vi "StepperControlWavelength.vi"() -> ()   [LabVIEW 2014, in "Stepper3D.lvlib"]
uses:
  stepper3D.lvlib
  <vilib>/Utility/error.llb/DialogType.ctl
  Enums/BoundaryStatus.ctl
  <vilib>/Utility/config.llb/Read Key (Double).vi
  <vilib>/Utility/config.llb/Write Key (Double).vi
  <vilib>/Utility/config.llb/NI_LVConfig.lvlib
  array.lib/Array.lvlib
panel:
  out "St3:Right":bool
  out "St3:Left":bool
  out "St2:Right":bool
  out "St2:Left":bool
  out "St1:Right":bool
  out "St1:Left":bool
  in  "Speed":string="300"
  in  "UI:LoadConversionTables":bool
  in  "Conversion 3":path=path "C:/Users/219-PC/Dropbox/МФД/Alexandr Bogomolov/Кумарин 47/Эталон.txt"
  in  "Conversion 2":path=path "C:/Users/219-PC/Dropbox/МФД/Alexandr Bogomolov/Кумарин 47/Эталон.txt"
  in  "Conversion 1":path=path "C:/Users/219-PC/Dropbox/МФД/Alexandr Bogomolov/Кумарин 47/Решетка 3D.txt"
  out "WL:WLToStepper3":dbl[][](array[numeric])
  out "WL:WLToStepper2":dbl[][](array[numeric])=[[115.0, 0.0], [135.0, 0.0]]
  out "WL:WLToStepper1":dbl[][](array[numeric])
  in  "WL:NewValue":dbl=450.0
  in  "WL:Stop":bool
  in  "WL:SetValue":bool
  out "App:RefreshLED":bool
  in  "App:RefreshRate":u32=500 caption="Refresh every"
  in  "App:Refresh":bool
  in  "App:Disconnect":bool
  in  "App:Connect":bool
  in  "St3:SetPos":bool
  in  "St2:SetPos":bool
  in  "St1:SetPos":bool
  in  "St:Stop":bool
  in  "St3:Steps":dbl
  in  "St3:NewPosition":dbl=2605.0
  out "St3:Position":dbl=2903.0
  in  "St2:Steps":dbl
  in  "St2:NewPosition":dbl=-2500.0
  out "St2:Position":dbl=-2500.0
  in  "St:DoSteps":bool
  in  "St1:Steps":dbl
  in  "St1:NewPosition":dbl=-57680.0
  out "St1:Position":dbl=-57680.0
  in  "App:ResourceName":refnum<visa-resource-name>="COM8"
  # "ms."
  # "BOUNDARY"
  # "FUNCTIONS"
  # "POSITION"
  # "NEW POSITION"
  # "STEPS"
  # "Решетка"
  # "Фабри-Перо"
  # "Кристалл"
  # "Длина волны"
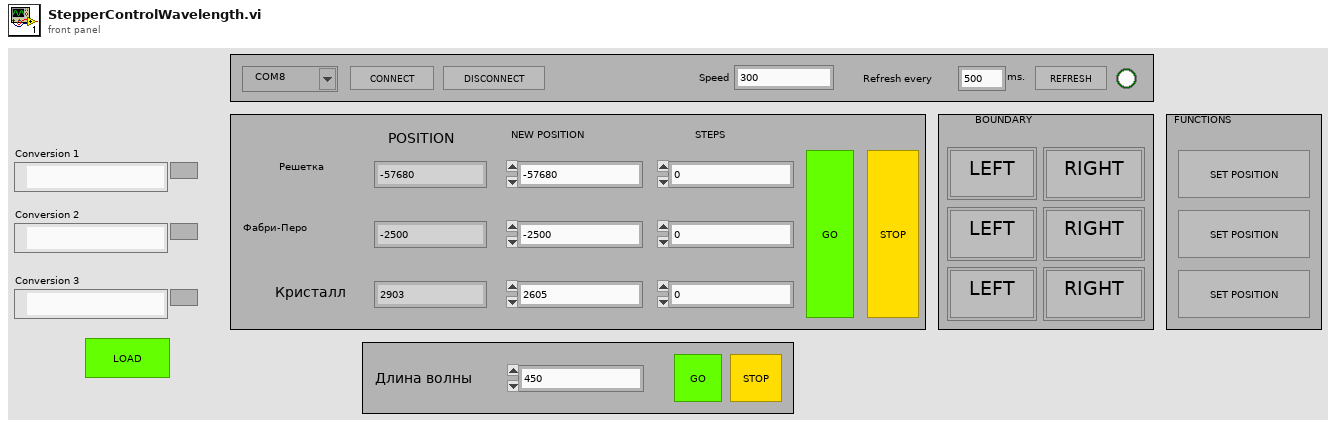
[diagram p1: front panel]
types:
  T1 = enum32{"invalid app kind", "Development System", "Run Time System", "Student Edition", "Embedded LabVIEW", "Evaluation", "Custom"}
  T2 = enum32{"Invalid", "Standard", "Closed", "Hidden", "Minimized", "Maximized"}
  T3 = typedef "stepper3D.lvlib/BoundaryStatus.ctl" = enum16{"NO BOUNDARY", "OUT OF LEFT", "OUT OF RIGHT"}
  T4 = cluster{"Core":cluster{"Current VI Reference":refnum<vi>, "Close Panel on Exit?":bool}, "VISA resource":refnum<visa-resource-name>, "App:RefreshRate":u32, "isConnected":bool, "appended path":path}
  T5 = typedef "DialogType.ctl" = u16
  T6 = cluster{"Current VI Reference":refnum<vi>, "Close Panel on Exit?":bool}
  T7 = typedef "NI_LVConfig.lvlib/Config Data RefNum.ctl" = refnum<k1>
  T8 = enum8{"Enabled", "Disabled", "Disabled and Grayed Out"}
  T9 = typedef "stepper3D.lvlib/CurrentStatus.ctl" = cluster{"desired":dbl[], "current":dbl[], "boundaries":T3[], "is running":bool}
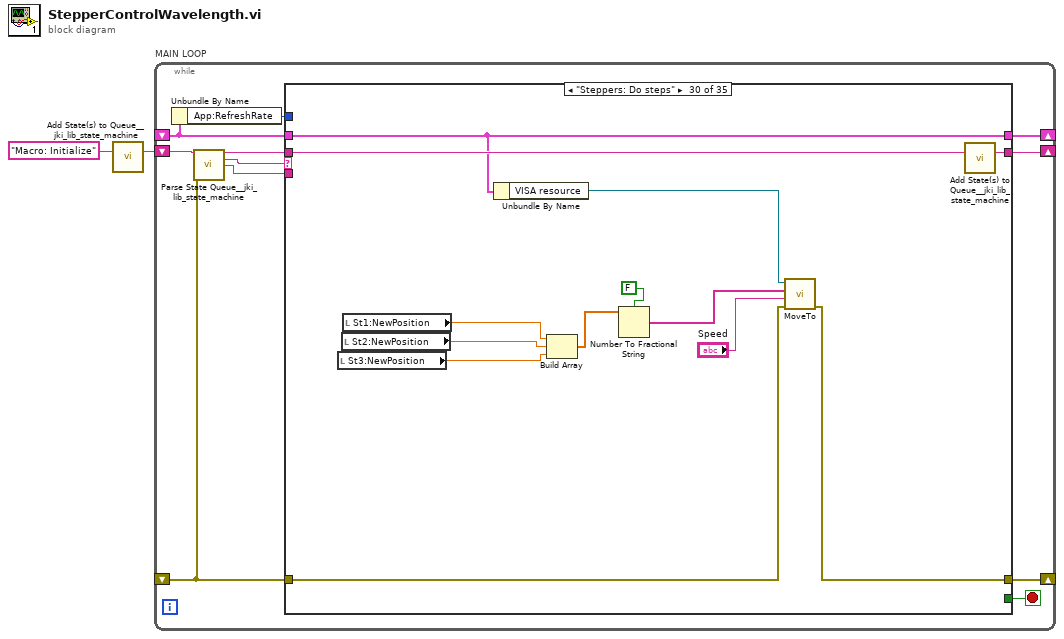
[diagram p0: block diagram]
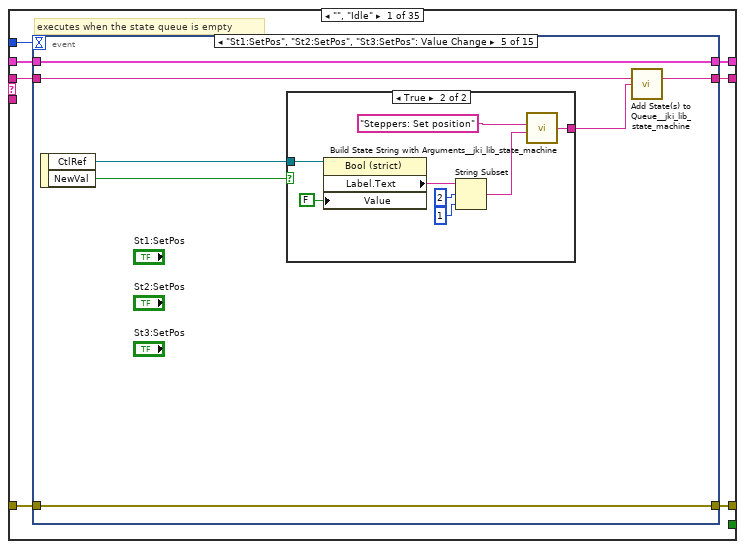
[diagram p2: hidden frame]
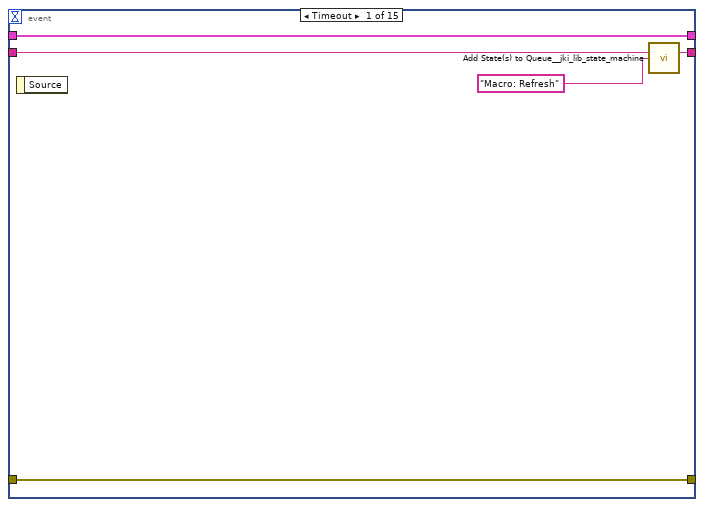
[diagram p3: hidden frame]
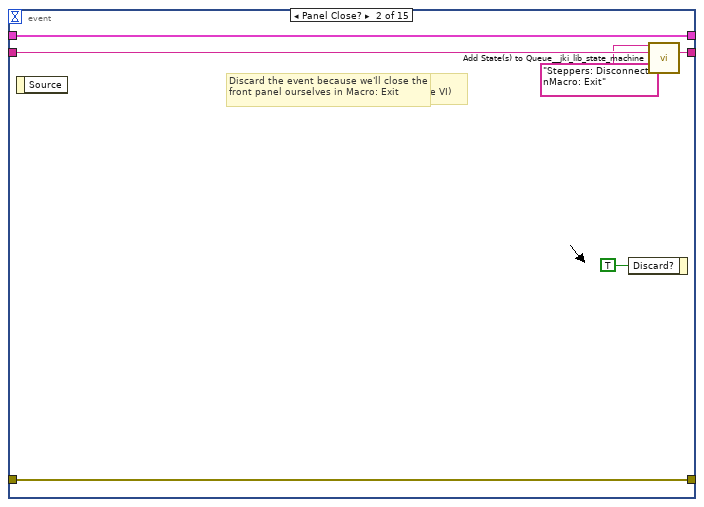
[diagram p4: hidden frame]
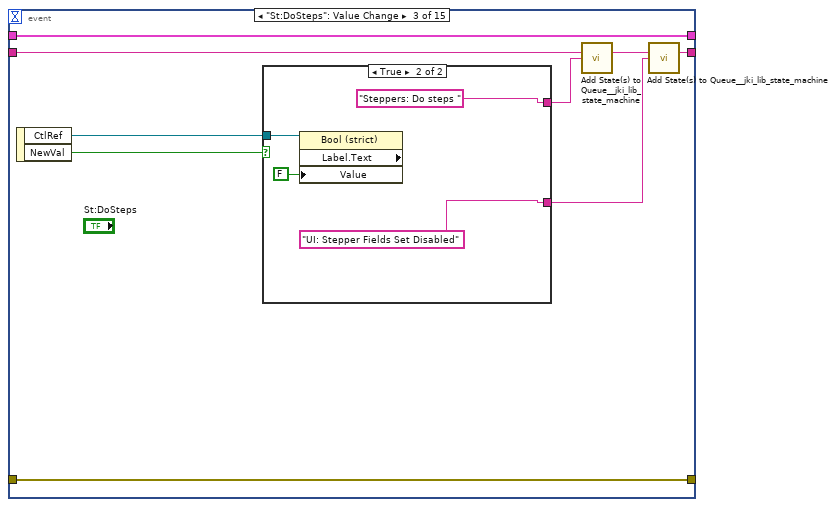
[diagram p5: hidden frame]
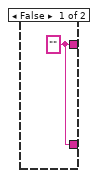
[diagram p6: hidden frame]
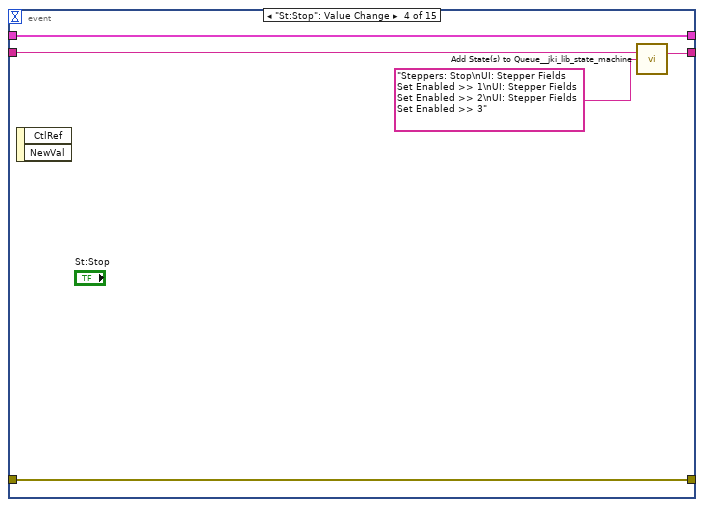
[diagram p7: hidden frame]
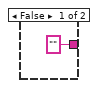
[diagram p8: hidden frame]
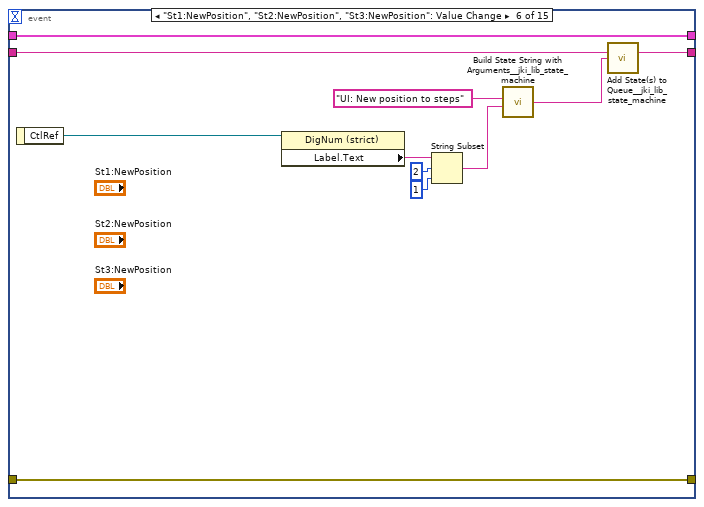
[diagram p9: hidden frame]
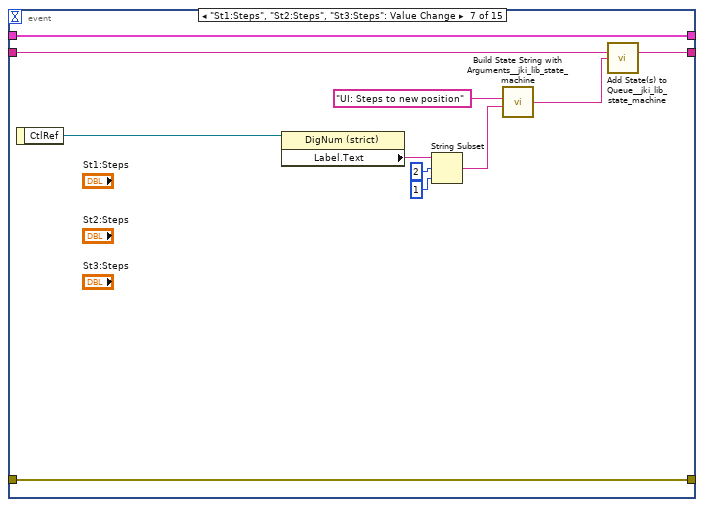
[diagram p10: hidden frame]
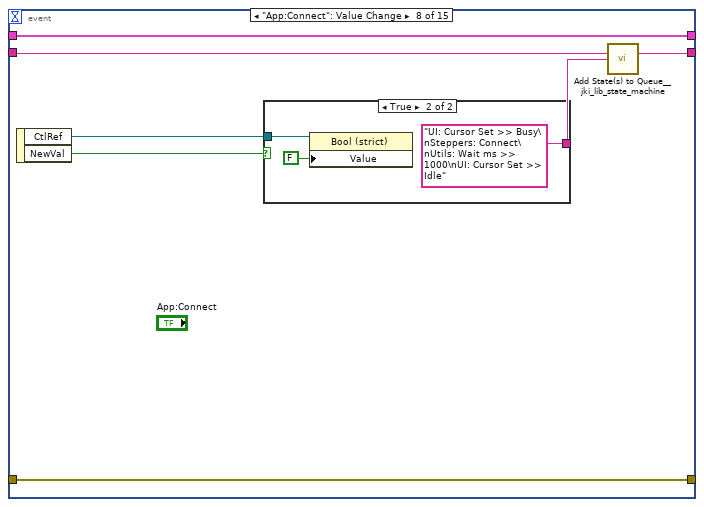
[diagram p11: hidden frame]
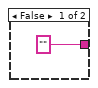
[diagram p12: hidden frame]
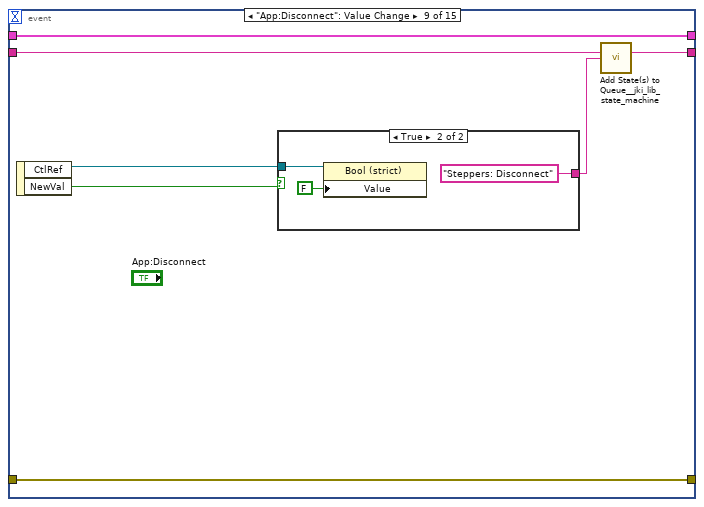
[diagram p13: hidden frame]
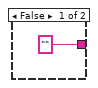
[diagram p14: hidden frame]
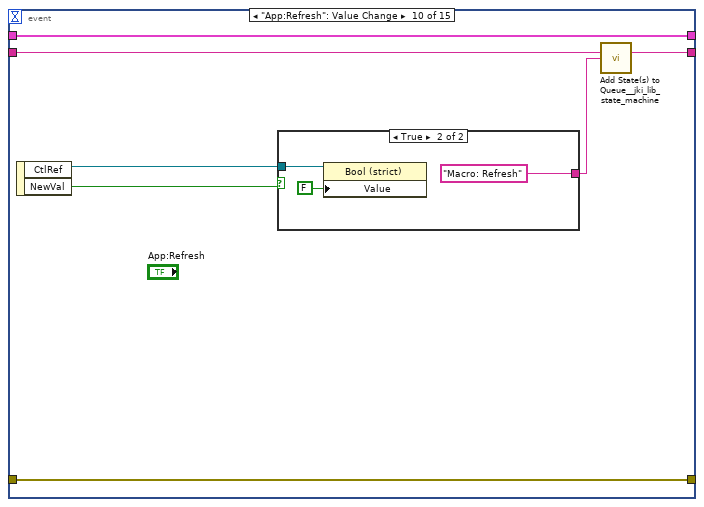
[diagram p15: hidden frame]
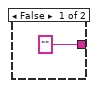
[diagram p16: hidden frame]
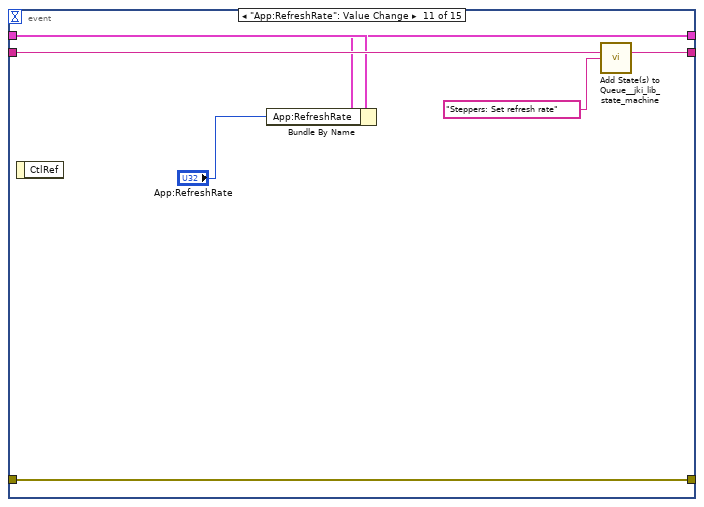
[diagram p17: hidden frame]
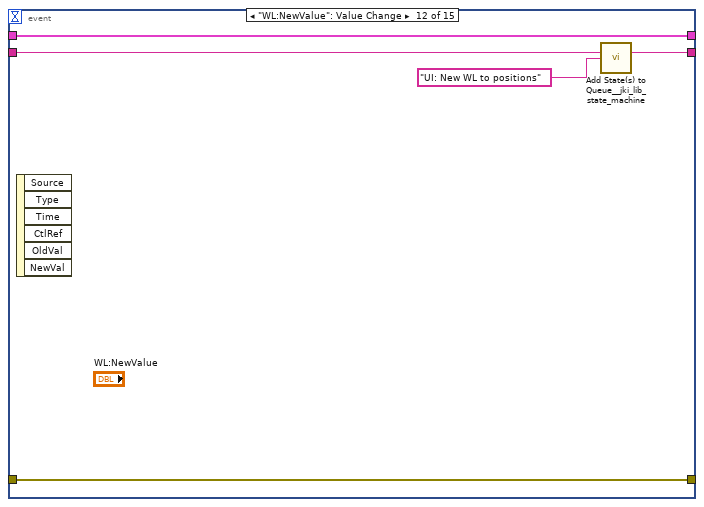
[diagram p18: hidden frame]
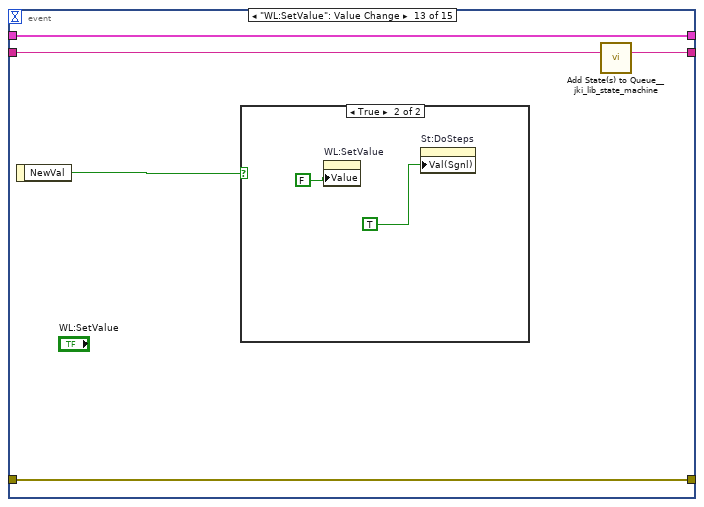
[diagram p19: hidden frame]
diagram:
  n1 = call <vilib>:"Add State(s) to Queue__jki_lib_state_machine.vi"("State(s) in (\"\")"="Macro: Initialize") -> ("States Out"=w2:string)  [unwired: 14 in]
  n2 = while "MAIN LOOP" {
    shift-right: [w7] -> _
    shift-left: _ -> [w3]
    shift-right: [w10] -> _
    shift-left: _ -> [w6]
    shift-right: [w9] -> _
    shift-left: w2 -> [w11]
    stop <- w8 stop-if-true
    n3 = Unbundle By Name(w3) -> ("App:RefreshRate"=w4:u32)
    n4 = call <vilib>:"Parse State Queue__jki_lib_state_machine.vi"("State Queue"=w11, "Error In (no error)"=w6) -> ("Remaining States"=w13:string, "Current State"=w5:string, "Arguments"=w12:string)  [unwired: 11 in]
    n5 = case shown="\"Steppers: Do steps\"" w5 {
      selector: w5 -> [_ _ w160 _ _ _ _ _ _ _ _ _ _ _ _ _ _ _ _ _ _ _ _ _ _ _ _ _ _ _ _ _ _ _ _]
      tunnel: w13 -> [w20 w159 w164 w182 w189 w194 w198 w209 w220 w239 w261 w267 w271 w276 w281 w286 w288 w307 w310 w328 w333 w340 w371 w376 w382 w394 w398 w404 w413 w429 w446 w457 w460 w527 w534]
      tunnel: w12 -> [_ _ _ _ _ _ _ _ _ _ _ _ _ _ _ _ w287 _ w311 w323 w336 w341 _ _ _ _ _ _ _ _ w442 _ _ _ w530]
      tunnel: w3 -> [w18 w156 w162 w173 w186 w192 w195 w206 _ w237 w258 w263 w268 w273 w278 w284 w290 w309 w313 w326 w337 w343 w368 w373 w379 w391 w395 w409 w412 w427 w443 w455 w465 w524 w531]
      tunnel: [w17 w157 w166 w179 errorcluster {"status"=FALSE, "code"=0, "source"=""} ("error out") w191 w196 w207 w217 w221 w259 w264 w269 w274 w279 w283 w289 w308 w312 w324 w335 w344 w369 w374 w380 w392 w396 w401 w414 w424 w441 w452 w462 w525 w532] -> w10
      tunnel: w6 -> [w16 w157 w165 w179 w185 w191 w196 w207 w217 w222 w259 w262 w269 w274 w279 w283 w289 w308 w312 w325 w335 w345 w369 w374 w380 w392 w396 w399 w415 w425 w440 w453 w463 w525 w532]
      tunnel: [w19 w158 w163 w181 w188 w193 w197 w208 w219 w238 w260 w266 w270 w275 w280 w285 w288 w307 w310 w327 w333 w340 w370 w375 w381 w393 w397 w405 w413 w428 w445 w456 w459 w526 w533] -> w9
      tunnel: [_ _ _ _ _ TRUE _ _ _ _ _ _ _ _ _ _ _ _ _ _ _ _ _ _ _ _ _ _ _ _ _ _ _ _ _] -> w8
      tunnel: [w15 w156 w162 w180 w186 w192 w195 w206 w218 w237 w258 w263 w268 w273 w278 w284 w290 w309 w313 w326 w337 w343 w368 w373 w379 w391 w395 w408 w411 w427 w443 w455 w465 w524 w531] -> w7
      tunnel: w4 -> [w14 _ _ _ _ _ _ _ _ _ _ _ _ _ _ _ _ _ _ _ _ _ _ _ _ _ _ _ _ _ _ _ _ _ _]
      frame "", "Idle" {
        # "executes when the state queue is empty"
        n6 = event shown="[4] \"St1:SetPos\", \"St2:SetPos\", \"St3:SetPos\": Value Change" {
          selector: _ -> [_ _ _ _ _ _ _ _ _ _ _ _ _ _ _]
          dyn-events: _ -> [_ _ _ _ _ _ _ _ _ _ _ _ _ _ _]
          timeout: w14 -> [_ _ _ _ _ _ _ _ _ _ _ _ _ _ _]
          tunnel: w20 -> [w25 w31 w36 w47 w53 w74 w85 w92 w102 w113 w127 w132 w137 w144 w152]
          tunnel: [w24 w30 w34 w48 w52 w73 w84 w93 w103 w114 w128 w133 w138 w145 w153] -> w19
          tunnel: w18 -> [w22 w28 w39 w50 w56 w76 w87 w94 w106 w117 w124 w130 w135 w142 w150]
          tunnel: [w23 w29 w38 w49 w55 w75 w86 w95 w100 w111 w125 w131 w136 w143 w151] -> w17
          tunnel: w16 -> [w23 w29 w38 w49 w55 w75 w86 w95 w100 w111 w125 w131 w136 w143 w151]
          tunnel: [w22 w28 w39 w50 w56 w76 w87 w94 w106 w117 w123 w130 w135 w142 w150] -> w15
          event Timeout {
            n7 = event-data() -> ()  [unwired: 1 in, 1 out]
            n8 = call <vilib>:"Add State(s) to Queue__jki_lib_state_machine.vi"("State(s) in (\"\")"=w25, "State(s) at Back (\"\")"="Macro: Refresh") -> ("States Out"=w24:string)  [unwired: 13 in]
          }
          event Panel Close? {
            # "Discard the event because we'll close the front panel ourselves in Macro: Exit"
            # "Close Panel button (pressed) Event\n(this executes Macro: Exit to terminate the VI)"
            n9 = event-data() -> ()  [unwired: 1 in, 1 out]
            n10 = event-data("Discard?"=TRUE) -> ()  [unwired: 1 in, 1 out]
            n11 = call <vilib>:"Add State(s) to Queue__jki_lib_state_machine.vi"("State(s) in Front (\"\")"="Steppers: Disconnect\nMacro: Exit", "State(s) in (\"\")"=w31) -> ("States Out"=w30:string)  [unwired: 13 in]
          }
          event "St:DoSteps": Value Change {
            n12 = event-data() -> ("CtlRef"=w40:refnum<vi>, "NewVal"=w37:bool)  [unwired: 1 in]
            n13 = case shown="True" w37 {
              tunnel: w40 -> [_ w45]
              tunnel: [w41 "Steppers: Do steps "] -> w35
              tunnel: [w41 "UI: Stepper Fields Set Disabled" ("State")] -> w32
              frame False {
                w41 = "" ("State with Arguments")
              }
              frame True {
                n14 = property class="Bool (strict)" props=["Label", "Text", "Value"](reference=w45, "Value"=FALSE) -> ()  [unwired: 1 in, 3 out]
              }
            }
            n15 = call <vilib>:"Add State(s) to Queue__jki_lib_state_machine.vi"("State(s) in (\"\")"=w36, "State(s) at Back (\"\")"=w35) -> ("States Out"=w33:string)  [unwired: 13 in]
            n16 = call <vilib>:"Add State(s) to Queue__jki_lib_state_machine.vi"("State(s) in (\"\")"=w33, "State(s) at Back (\"\")"=w32) -> ("States Out"=w34:string)  [unwired: 13 in]
          }
          event "St:Stop": Value Change {
            n17 = event-data() -> ()  [unwired: 1 in, 2 out]
            n18 = call <vilib>:"Add State(s) to Queue__jki_lib_state_machine.vi"("State(s) in (\"\")"=w47, "State(s) at Back (\"\")"="Steppers: Stop\nUI: Stepper Fields Set Enabled >> 1\nUI: Stepper Fields Set Enabled >> 2\nUI: Stepper Fields Set Enabled >> 3" ("State")) -> ("States Out"=w48:string)  [unwired: 13 in]
          }
          event "St1:SetPos", "St2:SetPos", "St3:SetPos": Value Change {
            n19 = event-data() -> ("CtlRef"=w57:refnum<vi>, "NewVal"=w54:bool)  [unwired: 1 in]
            n20 = case shown="True" w54 {
              tunnel: w57 -> [_ w66]
              tunnel: ["" ("State with Arguments") w60] -> w51
              frame False {
              }
              frame True {
                n21 = property class="Bool (strict)"(reference=w66, "Value"=FALSE) -> ("Label.Text"=w63:string)  [unwired: 1 in, 2 out]
                n22 = String Subset(string=w63, offset (0)=2, length (rest)=1 ("length (rest)")) -> (substring=w61:string)
                n23 = call <vilib>:"Build State String with Arguments__jki_lib_state_machine.vi"("Arguments (\"\")"=w61, "State"="Steppers: Set position") -> ("State with Arguments"=w60:string)  [unwired: 4 in]
              }
            }
            n24 = call <vilib>:"Add State(s) to Queue__jki_lib_state_machine.vi"("State(s) in (\"\")"=w53, "State(s) at Back (\"\")"=w51) -> ("States Out"=w52:string)  [unwired: 13 in]
          }
          event "St1:NewPosition", "St2:NewPosition", "St3:NewPosition": Value Change {
            n25 = event-data() -> ("CtlRef"=w77:refnum<vi>)  [unwired: 1 in]
            n26 = property class="DigNum (strict)"(reference=w77) -> ("Label.Text"=w69:string)  [unwired: 1 in, 2 out]
            n27 = String Subset(string=w69, offset (0)=2, length (rest)=1 ("length (rest)")) -> (substring=w67:string)
            n28 = call <vilib>:"Build State String with Arguments__jki_lib_state_machine.vi"("Arguments (\"\")"=w67, "State"="UI: New position to steps") -> ("State with Arguments"=w72:string)  [unwired: 4 in]
            n29 = call <vilib>:"Add State(s) to Queue__jki_lib_state_machine.vi"("State(s) in (\"\")"=w74, "State(s) at Back (\"\")"=w72) -> ("States Out"=w73:string)  [unwired: 13 in]
          }
          event "St1:Steps", "St2:Steps", "St3:Steps": Value Change {
            n30 = event-data() -> ("CtlRef"=w88:refnum<vi>)  [unwired: 1 in]
            n31 = property class="DigNum (strict)"(reference=w88) -> ("Label.Text"=w80:string)  [unwired: 1 in, 2 out]
            n32 = String Subset(string=w80, offset (0)=2, length (rest)=1 ("length (rest)")) -> (substring=w78:string)
            n33 = call <vilib>:"Build State String with Arguments__jki_lib_state_machine.vi"("Arguments (\"\")"=w78, "State"="UI: Steps to new position") -> ("State with Arguments"=w83:string)  [unwired: 4 in]
            n34 = call <vilib>:"Add State(s) to Queue__jki_lib_state_machine.vi"("State(s) in (\"\")"=w85, "State(s) at Back (\"\")"=w83) -> ("States Out"=w84:string)  [unwired: 13 in]
          }
          event "App:Connect": Value Change {
            n35 = event-data() -> ("CtlRef"=w91:refnum<vi>, "NewVal"=w90:bool)  [unwired: 1 in]
            n36 = case shown="True" w90 {
              tunnel: w91 -> [_ w99]
              tunnel: ["" "UI: Cursor Set >> Busy\nSteppers: Connect\nUtils: Wait ms >> 1000\nUI: Cursor Set >> Idle"] -> w89
              frame False {
              }
              frame True {
                n37 = property class="Bool (strict)"(reference=w99, "Value"=FALSE) -> ()  [unwired: 1 in, 2 out]
              }
            }
            n38 = call <vilib>:"Add State(s) to Queue__jki_lib_state_machine.vi"("State(s) in (\"\")"=w92, "State(s) at Back (\"\")"=w89) -> ("States Out"=w93:string)  [unwired: 13 in]
          }
          event "App:Disconnect": Value Change {
            n39 = event-data() -> ("CtlRef"=w105:refnum<vi>, "NewVal"=w104:bool)  [unwired: 1 in]
            n40 = case shown="True" w104 {
              tunnel: w105 -> [_ w110]
              tunnel: ["" "Steppers: Disconnect"] -> w101
              frame False {
              }
              frame True {
                n41 = property class="Bool (strict)"(reference=w110, "Value"=FALSE) -> ()  [unwired: 1 in, 2 out]
              }
            }
            n42 = call <vilib>:"Add State(s) to Queue__jki_lib_state_machine.vi"("State(s) in (\"\")"=w102, "State(s) at Back (\"\")"=w101) -> ("States Out"=w103:string)  [unwired: 13 in]
          }
          event "App:Refresh": Value Change {
            n43 = event-data() -> ("CtlRef"=w116:refnum<vi>, "NewVal"=w115:bool)  [unwired: 1 in]
            n44 = case shown="True" w115 {
              tunnel: w116 -> [_ w121]
              tunnel: ["" "Macro: Refresh"] -> w112
              frame False {
              }
              frame True {
                n45 = property class="Bool (strict)"(reference=w121, "Value"=FALSE) -> ()  [unwired: 1 in, 2 out]
              }
            }
            n46 = call <vilib>:"Add State(s) to Queue__jki_lib_state_machine.vi"("State(s) in (\"\")"=w113, "State(s) at Back (\"\")"=w112) -> ("States Out"=w114:string)  [unwired: 13 in]
          }
          event "App:RefreshRate": Value Change {
            n47 = event-data() -> ()  [unwired: 1 in, 1 out]
            n48 = Bundle By Name(cluster=w124, "App:RefreshRate"="App:RefreshRate") -> (w123:T4)
            n49 = call <vilib>:"Add State(s) to Queue__jki_lib_state_machine.vi"("State(s) in (\"\")"=w127, "State(s) at Back (\"\")"="Steppers: Set refresh rate") -> ("States Out"=w128:string)  [unwired: 13 in]
          }
          event "WL:NewValue": Value Change {
            n50 = event-data() -> ()  [unwired: 1 in, 6 out]
            n51 = call <vilib>:"Add State(s) to Queue__jki_lib_state_machine.vi"("State(s) in (\"\")"=w132, "State(s) at Back (\"\")"="UI: New WL to positions" ("State(s) at Back (\"\")")) -> ("States Out"=w133:string)  [unwired: 13 in]
          }
          event "WL:SetValue": Value Change {
            n52 = event-data() -> ("NewVal"=w134:bool)  [unwired: 1 in]
            n53 = case shown="True" w134 {
              frame False {
              }
              frame True {
                n54 = property on="WL:SetValue" class="Bool (strict)"("Value"=FALSE ("WL:SetValue")) -> ()  [unwired: 2 in, 2 out]
                n55 = property on="St:DoSteps" class="Bool (strict)"("Val(Sgnl)"=TRUE) -> ()  [unwired: 2 in, 2 out]
              }
            }
            n56 = call <vilib>:"Add State(s) to Queue__jki_lib_state_machine.vi"("State(s) in (\"\")"=w137) -> ("States Out"=w138:string)  [unwired: 14 in]
          }
          event "WL:Stop": Value Change {
            n57 = event-data() -> ("NewVal"=w141:bool)  [unwired: 1 in]
            n58 = case shown="True" w141 {
              frame False {
              }
              frame True {
                n59 = property on="WL:Stop" class="Bool (strict)"("Value"=FALSE ("WL:Stop")) -> ()  [unwired: 2 in, 2 out]
                n60 = property on="St:Stop" class="Bool (strict)"("Val(Sgnl)"=TRUE) -> ()  [unwired: 2 in, 2 out]
              }
            }
            n61 = call <vilib>:"Add State(s) to Queue__jki_lib_state_machine.vi"("State(s) in (\"\")"=w144) -> ("States Out"=w145:string)  [unwired: 14 in]
          }
          event "UI:LoadConversionTables": Value Change {
            n62 = event-data() -> ("NewVal"=w149:bool)  [unwired: 1 in]
            n63 = case shown="True" w149 {
              tunnel: [_ "Data: Load Conversion Files"] -> w148
              frame False {
              }
              frame True {
                n64 = property on="UI:LoadConversionTables" class="Bool (strict)"("Value"=FALSE) -> ()  [unwired: 2 in, 2 out]
              }
            }
            n65 = call <vilib>:"Add State(s) to Queue__jki_lib_state_machine.vi"("State(s) in (\"\")"=w152, "State(s) at Back (\"\")"=w148) -> ("States Out"=w153:string)  [unwired: 13 in]
          }
        }
      }
      frame "---------- Core ----------" {
        # "Do not put any code in this frame.\n(it is a separator no-op)"
        n66 = call <vilib>:"Add State(s) to Queue__jki_lib_state_machine.vi"("State(s) in (\"\")"=w159) -> ("States Out"=w158:string)  [unwired: 14 in]
      }
      frame Default {
        w169 = 42 items=["No error", "Argument error", "Memory is full", "Out of zone", "End of file", "File already open", "Generic file I/O error", "File not found", "File permission error", "Disk is full", "Duplicate path", "Too many files open", "System feature not enabled", "Resource file not found", "Cannot add resource", "Resource not found", "Image not found", "Image memory error", "Pen does not exist", "Config type invalid", "Config token not found", "Config parse error", "Config memory error", "Bad external code format", "Bad external code offset", "External code not present", "Null window", "Destroy window error", "Null menu", "Print aborted", "Bad print record", "Print driver error", "Windows error during printing", "Memory error during printing", "Print dialog error", "Generic print error", "Invalid device refnum", "Device not found", "Device parameter error", "Device unit error", "Cannot open device", "Device call aborted", "Generic error", "Cancelled by user", "Object ID too low", "Object ID too high", "Object not in heap", "Unknown heap", "Unknown object (invalid DefProc)", "Unknown object (DefProc not in table)", "Message out of range", "Invalid (null) method", "Unknown message", "Manager call not supported", "Bad address", "Network operation in progress", "Network operation timed out", "Connection is busy", "Network attribute not supported", "Network error", "Address in use", "System out of memory", "Connection aborted", "Connection refused", "Not connected", "Already connected", "Connection closed", "Initialization error (interapplication manager)", "Bad occurrence", "Wait on unbound occurrence handler", "Occurrence queue overflow", "Datalog type conflict", "Unused", "Unrecognized type (interapplication manager)", "Memory corrupt", "Failed to make temporary DLL", "Old CIN version", "Drag socket not found", "Failed to load drop-object", "Failed to register OLE object", "Failed to release OLE object", "Format specifier type mismatch", "Unknown format specifier", "Too few format specifiers", "Too many format specifiers", "Scan failed", "Newer CIN version", "Error converting to variant", "Runtime menu error", "Password tampered", "Variant attribute not found", "Incompatible variant data type", "Event data is not available", "Event Store is not present", "Occurrence is not found", "Event Queue is not created", "Event info is not available", "Refnum passed is NULL", "Error retrieving Class GUID", "Error retrieving CoClass GUID", "Error retrieving TypeLib GUID.", "Bad built application magic bytes.", "Specific driver is different from the specific driver associated with the Logical Name.", "There is no session opened to the class driver.", "Max Error", "MAX - Error with config objects", "MAX - Error loading configuration", "MAX - Group not supported"]
        # "Current State"
        # "Handle mistyped state name (developer tool)"
        n67 = Format Into String(format string="Software Exception: Unhandled State \"%s\"." ("message"), error in=w165, w160) -> (resulting string=w168:string, error out=w167:errorcluster)  [unwired: 1 in]
        n68 = call <vilib>:"Error Cluster From Error Code.vi"("show call chain? (False)"=TRUE, "error in (no error)"=w167, "error message (\"\")"=w168, "error code (0)"=w169) -> ("error out"=w166:errorcluster)  [unwired: 5 in]
        n69 = call <vilib>:"Add State(s) to Queue__jki_lib_state_machine.vi"("State(s) in (\"\")"=w164) -> ("States Out"=w163:string)  [unwired: 14 in]
      }
      frame "Initialize Core Data" {
        # "originally closed?"
        # "exe?"
        # "If panel starts closed or is an EXE, then close it when we exit"
        n70 = property class="VI"() -> ("Front Panel.Open"=w178:bool)  [unwired: 2 in, 2 out]
        n71 = property class="App"() -> ("App.Kind"=w177:T1)  [unwired: 2 in, 2 out]
        n72 = control-ref of="Current VI Reference"() -> (w171:refnum<vi>)
        n73 = Not(x=w178) -> (.not. x?=w175:bool)
        n74 = Equal?(x=w177, y=T1."Run Time System" ("Application:Kind")) -> (x = y?=w174:bool)
        n75 = Or(x=w175, y=w174) -> (x .or. y?=w172:bool)
        n76 = Bundle By Name(cluster=w173, "Core.Current VI Reference"=w171, "Core.Close Panel on Exit?"=w172) -> (w180:T4)
        n77 = call <vilib>:"Add State(s) to Queue__jki_lib_state_machine.vi"("State(s) in (\"\")"=w182) -> ("States Out"=w181:string)  [unwired: 14 in]
      }
      frame "Error Handler" {
        w183 = T5 2 items=["no dialog", "OK message", "continue or stop message", "OK message + warnings", "continue/stop + warnings"] ("type of dialog (OK msg:1)")
        # "Unhandled Error -- Display it"
        # "Handle any errors here.\nYou can also output any states to clean-up after errors occur"
        # "Clear error"
        n78 = call <vilib>:"General Error Handler.vi"("type of dialog (OK msg:1)"=w183, "error in (no error)"=w185) -> ()  [unwired: 9 in, 5 out]
        n79 = call <vilib>:"Add State(s) to Queue__jki_lib_state_machine.vi"("State(s) in Front (\"\")"="// Post Error States", "State(s) in (\"\")"=w189) -> ("States Out"=w188:string)  [unwired: 13 in]
      }
      frame "Exit" {
        n80 = call <vilib>:"Add State(s) to Queue__jki_lib_state_machine.vi"("State(s) in (\"\")"=w194) -> ("States Out"=w193:string)  [unwired: 14 in]
      }
      frame "---------- Data ----------" {
        # "Do not put any code in this frame.\n(It is a separator no-op. You can make a copy of this frame to create a new Data frame)"
        n81 = call <vilib>:"Add State(s) to Queue__jki_lib_state_machine.vi"("State(s) in (\"\")"=w198) -> ("States Out"=w197:string)  [unwired: 14 in]
      }
      frame "Data: Load Conversion Files" {
        n82 = call "readArrayFromFile.vi"("file"="Conversion 1") -> ("array"=→"WL:WLToStepper1":dbl[][])  [unwired: 1 in, 1 out]
        n83 = call "readArrayFromFile.vi"("file"="Conversion 2") -> ("array"=→"WL:WLToStepper2":dbl[][])  [unwired: 1 in, 1 out]
        n84 = call "readArrayFromFile.vi"("file"="Conversion 3") -> ("array"=→"WL:WLToStepper3":dbl[][])  [unwired: 1 in, 1 out]
        n85 = call <vilib>:"Add State(s) to Queue__jki_lib_state_machine.vi"("State(s) in (\"\")"=w209, "State(s) at Back (\"\")"="UI: New WL to positions" ("State(s) at Back (\"\")")) -> ("States Out"=w208:string)  [unwired: 13 in]
      }
      frame "Data: Initialize" {
        w214 = FALSE  # isConnected
        w215 = refnum<visa-resource-name> refnum  # VISA resource
        w216 = T6 {"Current VI Reference"=refnum, "Close Panel on Exit?"=FALSE}  # Core
        n86 = local read "App:RefreshRate"() -> (w213:u32)
        n87 = call <vilib>:"Application Directory.vi"() -> ("Application Directory"=w212:path)
        n88 = Build Path(base path=w212, name or relative path="steppers.config") -> (appended path=w210:path)
        n89 = Bundle("Core"=w216, "VISA resource"=w215, "App:RefreshRate"=w213, "isConnected"=w214, "appended path"=w210) -> (w218:T4)  [unwired: 1 in]
        n90 = call <vilib>:"Add State(s) to Queue__jki_lib_state_machine.vi"("State(s) in (\"\")"=w220) -> ("States Out"=w219:string)  [unwired: 14 in]
      }
      frame "Data: Read Config" {
        n91 = Unbundle By Name(w237) -> ("appended path"=w224:path)
        n92 = call <vilib>:"Open Config Data.vi"("error in (no error)"=w222, "configuration file path"=w224) -> ("error out"=w221:errorcluster, "refnum"=w223:T7)  [unwired: 7 in, 1 out]
        n93 = call-poly <vilib>:"Read Key.vi"("section"="current values", "key"="wavelength", "refnum"=w223) -> ("value"=w228:dbl)  [unwired: 5 in, 3 out]
        n94 = call-poly <vilib>:"Read Key.vi"("section"="current values", "key"="stepper1", "refnum"=w223) -> ("value"=w227:dbl)  [unwired: 5 in, 3 out]
        n95 = call-poly <vilib>:"Read Key.vi"("section"="current values", "key"="stepper2", "refnum"=w223) -> ("value"=w226:dbl)  [unwired: 5 in, 3 out]
        n96 = call-poly <vilib>:"Read Key.vi"("section"="current values", "key"="stepper3", "refnum"=w223) -> ("value"=w225:dbl)  [unwired: 5 in, 3 out]
        n97 = local write "WL:NewValue"(w228) -> ()
        n98 = local write "St1:NewPosition"(w227) -> ()
        n99 = local write "St2:NewPosition"(w226) -> ()
        n100 = local write "St3:NewPosition"(w225) -> ()
        n101 = call <vilib>:"Add State(s) to Queue__jki_lib_state_machine.vi"("State(s) in (\"\")"=w239) -> ("States Out"=w238:string)  [unwired: 14 in]
      }
      frame "Data: Write Config" {
        n102 = Unbundle By Name(w258) -> ("appended path"=w242:path)
        n103 = local read "St1:Position"() -> (w248:dbl)
        n104 = local read "WL:NewValue"() -> (w249:dbl)
        n105 = local read "St2:Position"() -> (w247:dbl)
        n106 = local read "St3:Position"() -> (w246:dbl)
        n107 = call <vilib>:"Open Config Data.vi"("configuration file path"=w242) -> ("refnum"=w241:T7)  [unwired: 8 in, 2 out]
        n108 = call-poly <vilib>:"Write Key.vi"("section"="current values", "value"=w249, "key"="wavelength", "refnum"=w241) -> ("refnum out"=w245:T7)  [unwired: 5 in, 2 out]
        n109 = call-poly <vilib>:"Write Key.vi"("section"="current values", "value"=w248, "key"="stepper1", "refnum"=w245) -> ("refnum out"=w244:T7)  [unwired: 5 in, 2 out]
        n110 = call-poly <vilib>:"Write Key.vi"("section"="current values", "value"=w247, "key"="stepper2", "refnum"=w244) -> ("refnum out"=w243:T7)  [unwired: 5 in, 2 out]
        n111 = call-poly <vilib>:"Write Key.vi"("section"="current values", "value"=w246, "key"="stepper3", "refnum"=w243) -> ("refnum out"=w240:T7)  [unwired: 5 in, 2 out]
        n112 = call <vilib>:"Close Config Data.vi"("refnum"=w240) -> ()  [unwired: 9 in, 2 out]
        n113 = call <vilib>:"Add State(s) to Queue__jki_lib_state_machine.vi"("State(s) in (\"\")"=w261) -> ("States Out"=w260:string)  [unwired: 14 in]
      }
      frame "Data: Cleanup" {
        n114 = Unbundle By Name(w263) -> ("Core.Current VI Reference"=w265:refnum<vi>)
        n115 = Close Reference(reference=w265, error in (no error)=w262) -> (error out=w264:errorcluster)
        n116 = call <vilib>:"Add State(s) to Queue__jki_lib_state_machine.vi"("State(s) in (\"\")"=w267) -> ("States Out"=w266:string)  [unwired: 14 in]
      }
      frame "---------- UI ----------" {
        # "Do not put any code in this frame.\n(It is a separator no-op. You can make a copy of this frame to create a new UI frame)"
        n117 = call <vilib>:"Add State(s) to Queue__jki_lib_state_machine.vi"("State(s) in (\"\")"=w271) -> ("States Out"=w270:string)  [unwired: 14 in]
      }
      frame "UI: Stepper Fields Set Enabled" {
        w272 = T8."Enabled" ("Disabled")
        # "Set Stepper Fields state .\n(Usage: \"UI: Stepper Fields Set Enabled >> 'Stepper Number'\")"
        n118 = property on="St1:NewPosition" class="DigNum (strict)"("DisabledEnum"=w272) -> ()  [unwired: 2 in, 2 out]
        n119 = property on="St2:NewPosition" class="DigNum (strict)"("DisabledEnum"=w272) -> ()  [unwired: 2 in, 2 out]
        n120 = property on="St1:Steps" class="DigNum (strict)"("DisabledEnum"=w272) -> ()  [unwired: 2 in, 2 out]
        n121 = property on="St2:Steps" class="DigNum (strict)"("DisabledEnum"=w272) -> ()  [unwired: 2 in, 2 out]
        n122 = property on="St3:NewPosition" class="DigNum (strict)"("DisabledEnum"=w272) -> ()  [unwired: 2 in, 2 out]
        n123 = property on="St3:Steps" class="DigNum (strict)"("DisabledEnum"=w272) -> ()  [unwired: 2 in, 2 out]
        n124 = property on="St:DoSteps" class="Bool (strict)"("DisabledEnum"=w272) -> ()  [unwired: 2 in, 2 out]
        n125 = call <vilib>:"Add State(s) to Queue__jki_lib_state_machine.vi"("State(s) in (\"\")"=w276) -> ("States Out"=w275:string)  [unwired: 14 in]
      }
      frame "UI: Stepper Fields Set Disabled" {
        w277 = T8."Disabled and Grayed Out" ("Disabled")
        # "Set Stepper Fields state .\n(Usage: \"UI: Stepper Fields Set Enabled >> 'Stepper Number'\")"
        n126 = property on="St1:NewPosition" class="DigNum (strict)"("DisabledEnum"=w277) -> ()  [unwired: 2 in, 2 out]
        n127 = property on="St1:Steps" class="DigNum (strict)"("DisabledEnum"=w277) -> ()  [unwired: 2 in, 2 out]
        n128 = property on="St2:NewPosition" class="DigNum (strict)"("DisabledEnum"=w277) -> ()  [unwired: 2 in, 2 out]
        n129 = property on="St2:Steps" class="DigNum (strict)"("DisabledEnum"=w277) -> ()  [unwired: 2 in, 2 out]
        n130 = property on="St3:NewPosition" class="DigNum (strict)"("DisabledEnum"=w277) -> ()  [unwired: 2 in, 2 out]
        n131 = property on="St3:Steps" class="DigNum (strict)"("DisabledEnum"=w277) -> ()  [unwired: 2 in, 2 out]
        n132 = property on="St:DoSteps" class="Bool (strict)"("DisabledEnum"=w277) -> ()  [unwired: 2 in, 2 out]
        n133 = call <vilib>:"Add State(s) to Queue__jki_lib_state_machine.vi"("State(s) in (\"\")"=w281) -> ("States Out"=w280:string)  [unwired: 14 in]
      }
      frame "UI: Initialize" {
        n134 = call <vilib>:"Add State(s) to Queue__jki_lib_state_machine.vi"("State(s) in Front (\"\")"="UI: Stepper Fields Set Enabled" ("State(s) in Front (\"\")"), "State(s) in (\"\")"=w286) -> ("States Out"=w285:string)  [unwired: 13 in]
      }
      frame "UI: Steps to new position" {
        n135 = case shown="\"3\"" w287 {
          frame "1" {
            n136 = local read "St1:Position"() -> (w293:dbl)
            n137 = local read "St1:Steps"() -> (w292:dbl)
            n138 = Add(x=w293, y=w292) -> (x+y=w291:dbl)
            n139 = local write "St1:NewPosition"(w291) -> ()
          }
          frame "2" {
            n140 = local read "St2:Position"() -> (w296:dbl)
            n141 = local read "St2:Steps"() -> (w295:dbl)
            n142 = Add(x=w296, y=w295) -> (x+y=w294:dbl)
            n143 = local write "St2:NewPosition"(w294) -> ()
          }
          frame "3" {
            n144 = local read "St3:Position"() -> (w299:dbl)
            n145 = local read "St3:Steps"() -> (w298:dbl)
            n146 = Add(x=w299, y=w298) -> (x+y=w297:dbl)
            n147 = local write "St3:NewPosition"(w297) -> ()
          }
          frame Default {
          }
        }
      }
      frame "UI: New WL to positions" {
        n148 = local read "WL:WLToStepper1"() -> (w306:dbl[][])
        n149 = local read "WL:WLToStepper2"() -> (w304:dbl[][])
        n150 = local read "WL:WLToStepper3"() -> (w305:dbl[][])
        n151 = property on="WL:NewValue" class="DigNum (strict)"() -> ("Value"=w300:dbl)  [unwired: 2 in, 2 out]
        n152 = call "GetNearestValue.vi"("Value"=w300, "Array"=w306) -> ("Nearest Value"=w303:dbl)  [unwired: 9 in]
        n153 = call "GetNearestValue.vi"("Value"=w300, "Array"=w304) -> ("Nearest Value"=w302:dbl)  [unwired: 9 in]
        n154 = call "GetNearestValue.vi"("Value"=w300, "Array"=w305) -> ("Nearest Value"=w301:dbl)  [unwired: 9 in]
        n155 = property on="St1:NewPosition" class="DigNum (strict)"("Val(Sgnl)"=w303) -> ()  [unwired: 2 in, 2 out]
        n156 = property on="St2:NewPosition" class="DigNum (strict)"("Val(Sgnl)"=w302) -> ()  [unwired: 2 in, 2 out]
        n157 = property on="St3:NewPosition" class="DigNum (strict)"("Val(Sgnl)"=w301) -> ()  [unwired: 2 in, 2 out]
      }
      frame "UI: New position to steps" {
        n158 = case shown="Default" w311 {
          frame Default {
          }
          frame "1" {
            n159 = local read "St1:NewPosition"() -> (w316:dbl)
            n160 = local read "St1:Position"() -> (w315:dbl)
            n161 = Subtract(x=w316, y=w315) -> (x-y=w314:dbl)
            n162 = local write "St1:Steps"(w314) -> ()
          }
          frame "2" {
            n163 = local read "St2:NewPosition"() -> (w319:dbl)
            n164 = local read "St2:Position"() -> (w318:dbl)
            n165 = Subtract(x=w319, y=w318) -> (x-y=w317:dbl)
            n166 = local write "St2:Steps"(w317) -> ()
          }
          frame "3" {
            n167 = local read "St3:NewPosition"() -> (w322:dbl)
            n168 = local read "St3:Position"() -> (w321:dbl)
            n169 = Subtract(x=w322, y=w321) -> (x-y=w320:dbl)
            n170 = local write "St3:Steps"(w320) -> ()
          }
        }
      }
      frame "UI: Cursor Set" {
        # "Argument"
        # "Set and Unset Cursor Busy.\n(Usage: \"UI: Cursor Set >> Busy|Idle\")"
        n171 = case shown="\"Idle\", Default" w323 {
          tunnel: w325 -> [w330 w332]
          tunnel: [w329 w331] -> w324
          frame "Idle", Default {
            n172 = call <vilib>:"Unset Busy.vi"("error in (no error)"=w330) -> ("error out"=w329:errorcluster)  [unwired: 10 in]
          }
          frame "Busy" {
            n173 = call <vilib>:"Set Busy.vi"("error in (no error)"=w332) -> ("error out"=w331:errorcluster)  [unwired: 9 in, 1 out]
          }
        }
        n174 = call <vilib>:"Add State(s) to Queue__jki_lib_state_machine.vi"("State(s) in (\"\")"=w328) -> ("States Out"=w327:string)  [unwired: 14 in]
      }
      frame "UI: RefreshLED Set" {
        # "Argument"
        # "Set and Unset RefreshLED.\n(Usage: \"UI: RefreshLED Set >> On|Off\")"
        n175 = case shown="\"Off\", Default" w336 {
          tunnel: [TRUE FALSE] -> w334
          frame "On" {
          }
          frame "Off", Default {
          }
        }
        "App:RefreshLED" <- w334
      }
      frame "UI: Front Panel State" {
        # "Argument"
        # "Set Front Panel Open or Closed\n(Usage: \"UI: Front Panel State >> Open|Close\")"
        n176 = Unbundle By Name(w343) -> ("Core.Current VI Reference"=w342:refnum<vi>)
        n177 = case shown="\"Open\", Default" w341 {
          tunnel: w345 -> [w349 w362]
          tunnel: [w351 w363] -> w344
          tunnel: w342 -> [w350 w360]
          frame "Open", Default {
            n178 = property class="VI"(reference=w350, error in=w349) -> (reference out=w347:refnum<vi>, error out=w348:errorcluster, "Front Panel.Open"=w346:bool)
            n179 = case shown="True" w346 {
              tunnel: [w354 w357] -> w351
              tunnel: w348 -> [w353 w357]
              tunnel: w347 -> [w352 _]
              frame False {
                n180 = invoke class="VI" method="FP.Open"(reference=w352, error in=w353, "Activate"=TRUE, "State"=T2."Standard") -> (error out=w354:errorcluster)  [unwired: 1 in, 4 out]
              }
              frame True {
              }
            }
          }
          frame "Close" {
            n181 = property class="VI"(reference=w360, error in=w362) -> (reference out=w359:refnum<vi>, error out=w361:errorcluster, "Front Panel.Open"=w358:bool)
            n182 = case shown="True" w358 {
              tunnel: [w364 w367] -> w363
              tunnel: w361 -> [w364 w366]
              tunnel: w359 -> [_ w365]
              frame False {
              }
              frame True {
                n183 = invoke class="VI" method="FP.Close"(reference=w365, error in=w366) -> (error out=w367:errorcluster)  [unwired: 1 in, 2 out]
              }
            }
          }
        }
      }
      frame "---------- Macro ----------" {
        # "Do not put any code in this frame.\n(It is a separator no-op. You can make a copy of this frame to create a new Macro frame)"
        n184 = call <vilib>:"Add State(s) to Queue__jki_lib_state_machine.vi"("State(s) in (\"\")"=w371) -> ("States Out"=w370:string)  [unwired: 14 in]
      }
      frame "Macro: Initialize" {
        w372 = "Data: Initialize\nInitialize Core Data\nUI: Initialize\nUI: Front Panel State >> Open\nData: Load Conversion Files\nData: Read Config\nSteppers: Connect"  # Data: Initialize Initialize Core Data UI: Initialize UI: Front Panel State >> Open Data: Load Conversion Files Data: Read Config Steppers: Connect
        # "Initialization Macro\n(This is called once, when the VI starts)"
        n185 = call <vilib>:"Add State(s) to Queue__jki_lib_state_machine.vi"("State(s) in Front (\"\")"=w372, "State(s) in (\"\")"=w376) -> ("States Out"=w375:string)  [unwired: 13 in]
      }
      frame "Macro: Refresh" {
        n186 = Unbundle By Name(w379) -> ("isConnected"=w378:bool)
        n187 = case shown="True" w378 {
          tunnel: ["" "UI: RefreshLED Set >> On\nSteppers: Refresh\nUI: RefreshLED Set >> Off"] -> w377
          frame False {
          }
          frame True {
          }
        }
        n188 = call <vilib>:"Add State(s) to Queue__jki_lib_state_machine.vi"("State(s) in Front (\"\")"=w377, "State(s) in (\"\")"=w382) -> ("States Out"=w381:string)  [unwired: 13 in]
      }
      frame "Macro: Exit" {
        # "Exit Macro\n(This is called once, when the VI exits)"
        n189 = Unbundle By Name(w391) -> ("Core.Close Panel on Exit?"=w390:bool)
        n190 = Select(t="UI: Front Panel State >> Close", s=w390, f="") -> (s? t:f=w387:string)
        n191 = call <vilib>:"Add State(s) to Queue__jki_lib_state_machine.vi"("State(s) in (\"\")"=w387, "State(s) at Back (\"\")"="Steppers: Disconnect\nData: Cleanup\nExit") -> ("States Out"=w385:string)  [unwired: 13 in]
        n192 = call <vilib>:"Add State(s) to Queue__jki_lib_state_machine.vi"("State(s) in Front (\"\")"=w385, "State(s) in (\"\")"=w394) -> ("States Out"=w393:string)  [unwired: 13 in]
      }
      frame "---------- Steppers ----------" {
        # "Template Separator\n(You can make a copy of, or modify, this frame)"
        n193 = call <vilib>:"Add State(s) to Queue__jki_lib_state_machine.vi"("State(s) in (\"\")"=w398) -> ("States Out"=w397:string)  [unwired: 14 in]
      }
      frame "Steppers: Connect" {
        # "Connect to steppers"
        n194 = call "connect.vi"("error in"=w399, "VISA resource name"="App:ResourceName") -> ("error out"=w401:errorcluster, "VISA resource name out"=w400:refnum<visa-resource-name>)
        n195 = Unbundle By Name(w401) -> ("status"=w406:bool)
        n196 = Not(x=w406) -> (.not. x?=w407:bool)
        n197 = Bundle By Name(cluster=w409, "isConnected"=w407, "VISA resource"=w400) -> (w408:T4)
        n198 = call <vilib>:"Add State(s) to Queue__jki_lib_state_machine.vi"("State(s) in Front (\"\")"="Macro: Refresh\nSteppers: Set position >> 1\nSteppers: Set position >> 2\nSteppers: Set position >> 3" ("State(s) at Back (\"\")"), "State(s) in (\"\")"=w404) -> ("States Out"=w405:string)  [unwired: 13 in]
      }
      frame "Steppers: Disconnect" {
        n199 = Unbundle By Name(w412) -> ("VISA resource"=w416:refnum<visa-resource-name>)
        n200 = call "disconnect.vi"("error in"=w415, "VISA resource name"=w416) -> ("error out"=w414:errorcluster)  [unwired: 1 in]
        n201 = Bundle By Name(cluster=w412, "isConnected"=FALSE) -> (w411:T4)
      }
      frame "Steppers: Do steps" {
        n202 = local read "St3:NewPosition"() -> (w420:dbl)
        n203 = local read "St2:NewPosition"() -> (w421:dbl)
        n204 = local read "St1:NewPosition"() -> (w422:dbl)
        n205 = Unbundle By Name(w427) -> ("VISA resource"=w426:refnum<visa-resource-name>)
        n206 = Build Array(w422, w421, w420) -> (w418:dbl[])
        n207 = Number To Fractional String(use system decimal point (T)=FALSE, number=w418) -> (F-format string=w417:string[])  [unwired: 2 in]
        n208 = call "MoveTo.vi"("error in (no error)"=w425, "speed"="Speed", "positions"=w417, "VISA Refnum in"=w426) -> ("error out"=w424:errorcluster)  [unwired: 6 in, 1 out]
        n209 = call <vilib>:"Add State(s) to Queue__jki_lib_state_machine.vi"("State(s) in (\"\")"=w429) -> ("States Out"=w428:string)  [unwired: 14 in]
      }
      frame "Steppers: Set position" {
        w438 = ""
        n210 = case shown="\"1\"" w442 {
          tunnel: [0 ("St3:Steps") w448 w449 w450] -> w432
          frame Default {
          }
          frame "1" {
            n211 = local read "St1:NewPosition"() -> (w448:dbl)
          }
          frame "2" {
            n212 = local read "St2:NewPosition"() -> (w449:dbl)
          }
          frame "3" {
            n213 = local read "St3:NewPosition"() -> (w450:dbl)
          }
        }
        n214 = Decimal String To Number(string=w442, default (0L)=u16 0 ("default (0 I32)")) -> (number=w436:u16)  [unwired: 1 in, 1 out]
        n215 = Decrement(x=w436) -> (x-1=w435:u16)
        n216 = Build Array(w438, w438, w438) -> (w437:string[])
        n217 = Unbundle By Name(w443) -> ("VISA resource"=w439:refnum<visa-resource-name>)
        n218 = Number To Fractional String(use system decimal point (T)=FALSE, number=w432) -> (F-format string=w431:string)  [unwired: 2 in]
        n219 = Replace Array Subset(array=w437, new element=w431, index=w435) -> (w434:string[])
        n220 = call "SetPosition.vi"("error in (no error)"=w440, "positions"=w434, "VISA Refnum in"=w439) -> ("error out"=w441:errorcluster)  [unwired: 7 in, 1 out]
        n221 = call <vilib>:"Add State(s) to Queue__jki_lib_state_machine.vi"("State(s) in (\"\")"=w446, "State(s) at Back (\"\")"="Data: Write Config" ("State(s) at Back (\"\")")) -> ("States Out"=w445:string)  [unwired: 13 in]
      }
      frame "Steppers: Stop" {
        n222 = Unbundle By Name(w455) -> ("VISA resource"=w454:refnum<visa-resource-name>)
        n223 = call "Stop.vi"("error in (no error)"=w453, "VISA Refnum in"=w454) -> ("error out"=w452:errorcluster)  [unwired: 8 in, 1 out]
        n224 = call <vilib>:"Add State(s) to Queue__jki_lib_state_machine.vi"("State(s) in (\"\")"=w457, "State(s) at Back (\"\")"="Data: Write Config" ("State(s) at Back (\"\")")) -> ("States Out"=w456:string)  [unwired: 13 in]
      }
      frame "Steppers: Refresh" {
        n225 = Unbundle By Name(w465) -> ("VISA resource"=w464:refnum<visa-resource-name>, "isConnected"=w461:bool)
        n226 = case shown="True" w461 {
          tunnel: w464 -> [_ w471]
          tunnel: w463 -> [w466 w472]
          tunnel: [w466 w473] -> w462
          frame False {
          }
          frame True {
            n227 = call "GetCurrentStatus.vi"("error in (no error)"=w472, "VISA Refnum in"=w471) -> ("error out"=w473:errorcluster, "status"=w474:T9)  [unwired: 7 in, 1 out]
            n228 = Unbundle By Name(w474) -> ("current"=w475:dbl[], "boundaries"=w470:T3[], "is running"=w467:bool)
            n229 = case shown="False" w467 {
              frame False {
                n230 = property on="St:Stop" class="Bool (strict)"("Val(Sgnl)"=TRUE) -> ()  [unwired: 2 in, 2 out]
              }
              frame True {
              }
            }
            n231 = for {
              tunnel: w475 -> [w482] mode=indexing
              tunnel: w470 -> [w479] mode=indexing
              tunnel: BoundaryStatus."NO BOUNDARY" ("Enum") -> [w477]
              tunnel: BoundaryStatus."OUT OF LEFT" ("Enum") -> [w480]
              i -> [w484]
              n232 = Not Equal?(x=w479, y=w477) -> (x != y?=w481:bool)
              n233 = Increment(x=w484) -> (x+1=w483:i32)
              n234 = Equal?(x=w479, y=w480) -> (x = y?=w478:bool)
              n235 = case shown="3" w483 {
                tunnel: w482 -> [_ w489 w502 w515]
                tunnel: w479 -> [_ _ _ _]
                tunnel: w481 -> [_ w488 w501 w514]
                tunnel: w478 -> [_ w487 w500 w513]
                frame Default {
                }
                frame 1 {
                  n236 = case shown="True" w488 {
                    tunnel: w487 -> [_ w493]
                    tunnel: [w490 w492] -> w486
                    tunnel: [w490 w491] -> w485
                    frame False {
                      w490 = FALSE
                    }
                    frame True {
                      n237 = case shown="False" w493 {
                        tunnel: [FALSE TRUE] -> w492
                        tunnel: [TRUE FALSE] -> w491
                        frame False {
                        }
                        frame True {
                        }
                      }
                    }
                  }
                  "St1:Right" <- w485
                  "St1:Left" <- w486
                  "St1:Position" <- w489
                }
                frame 2 {
                  n238 = case shown="False" w501 {
                    tunnel: w500 -> [_ w506]
                    tunnel: [w503 w505] -> w499
                    tunnel: [w503 w504] -> w498
                    frame False {
                      w503 = FALSE
                    }
                    frame True {
                      n239 = case shown="False" w506 {
                        tunnel: [FALSE TRUE] -> w505
                        tunnel: [TRUE FALSE] -> w504
                        frame False {
                        }
                        frame True {
                        }
                      }
                    }
                  }
                  "St2:Left" <- w499
                  "St2:Right" <- w498
                  "St2:Position" <- w502
                }
                frame 3 {
                  n240 = case shown="True" w514 {
                    tunnel: w513 -> [_ w519]
                    tunnel: [w516 w518] -> w511
                    tunnel: [w516 w517] -> w512
                    frame False {
                      w516 = FALSE
                    }
                    frame True {
                      n241 = case shown="True" w519 {
                        tunnel: [FALSE TRUE] -> w518
                        tunnel: [TRUE FALSE] -> w517
                        frame False {
                        }
                        frame True {
                        }
                      }
                    }
                  }
                  "St3:Left" <- w511
                  "St3:Right" <- w512
                  "St3:Position" <- w515
                }
              }
            }
          }
        }
        n242 = call <vilib>:"Add State(s) to Queue__jki_lib_state_machine.vi"("State(s) in Front (\"\")"="UI: New position to steps >> 1\nUI: New position to steps >> 2\nUI: New position to steps >> 3\nData: Write Config" ("State(s) at Back (\"\")"), "State(s) in (\"\")"=w460) -> ("States Out"=w459:string)  [unwired: 13 in]
      }
      frame "---------- Utils ---------" {
        # "Template Separator\n(You can make a copy of, or modify, this frame)"
        n243 = call <vilib>:"Add State(s) to Queue__jki_lib_state_machine.vi"("State(s) in (\"\")"=w527) -> ("States Out"=w526:string)  [unwired: 14 in]
      }
      frame "Utils: Wait ms" {
        # "Wait ms >> \"number of ms\""
        n244 = Decimal String To Number(string=w530, default (0L)=u32 0 ("default (0 I32)")) -> (number=w529:u32)  [unwired: 1 in, 1 out]
        n245 = Wait (ms)(milliseconds to wait=w529) -> ()  [unwired: 1 out]
        n246 = call <vilib>:"Add State(s) to Queue__jki_lib_state_machine.vi"("State(s) in (\"\")"=w534) -> ("States Out"=w533:string)  [unwired: 14 in]
      }
    }
  }
